vi "Read Next PNG Chunk.vi"(8 "error in (no error)":errorcluster, 11 "Byte Stream File in":refnum<file>) -> (0 "error out":errorcluster, 1 "data":u8[](array[numeric]), 2 "Type":string, 3 "Byte Stream File out":refnum<file>, 4 "CRC":u32, 5 "Length":u32)   [LabVIEW 2021, in "Files.lvlib"]
uses:
  Files.lvlib
  93311296-cc19-459f-8a29-a5908e25dff8.vi
  d1c91a06-6000-4e7e-a644-8d6add85a8ab.vi
  93311296-cc19-459f-8a29-a5908e25dff8.vi/539bd7ec-d9e8-460f-a56d-a449b4a86a5e.vi
  d1c91a06-6000-4e7e-a644-8d6add85a8ab.vi/539bd7ec-d9e8-460f-a56d-a449b4a86a5e.vi
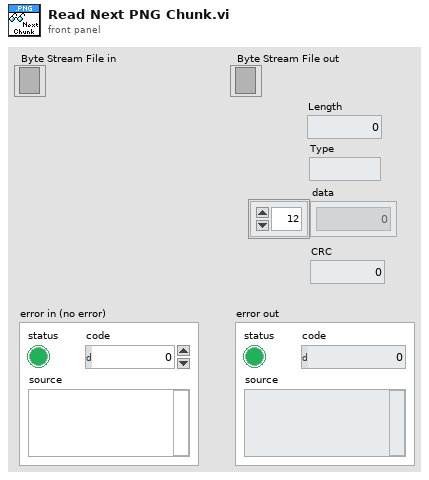
[diagram p1: front panel]
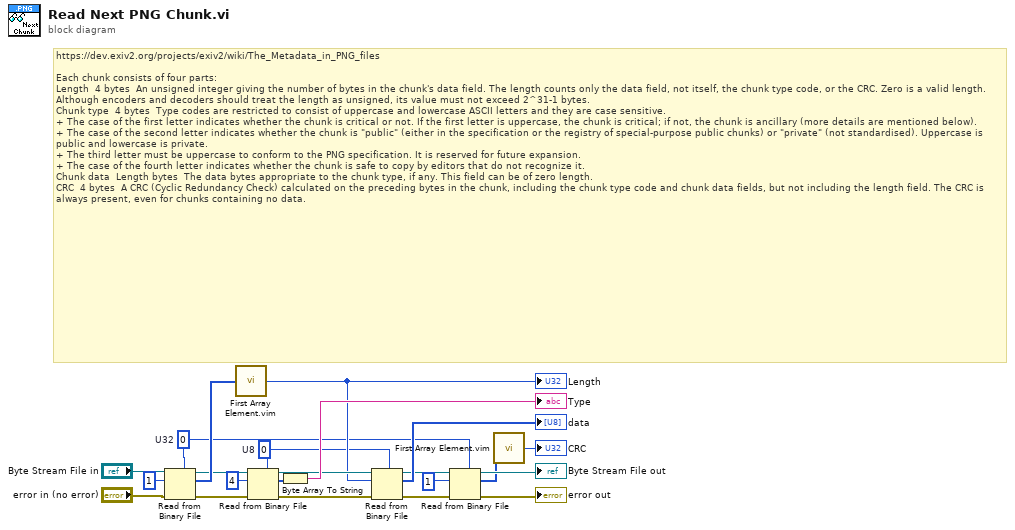
[diagram p0: block diagram]
diagram:
  w9 = u8 0  # U8
  w3 = u32 0  # U32
  # "https://dev.exiv2.org/projects/exiv2/wiki/The_Metadata_in_PNG_files\n\nEach chunk consists of four parts:\nLength \t4 bytes \tAn unsigned integer giving the number of bytes in the chunk's data field. The length counts only the data field, not itself, the chunk type code, or the CRC. Zero is a valid length. Although encoders and decoders should treat the length as unsigned, its value must not exceed 2^31-1 bytes.\nChunk type \t4 bytes \tType codes are restricted to consist of uppercase and lowercase ASCII letters and they are case sensitive.\n+ The case of the first letter indicates whether the chunk is critical or not. If the first letter is uppercase, the chunk is critical; if not, the chunk is ancillary (more details are mentioned below).\n+ The case of the second letter indicates whether the chunk is \"public\" (either in the specification or the registry of special-purpose public chunks) or \"private\" (not standardised). Uppercase is public and lowercase is private.\n+ The third letter must be uppercase to conform to the PNG specification. It is reserved for future expansion.\n+ The case of the fourth letter indicates whether the chunk is safe to copy by editors that do not recognize it.\nChunk data \tLength bytes \tThe data bytes appropriate to the chunk type, if any. This field can be of zero length.\nCRC \t4 bytes \tA CRC (Cyclic Redundancy Check) calculated on the preceding bytes in the chunk, including the chunk type code and chunk data fields, but not including the length field. The CRC is always present, even for chunks containing no data."
  n1 = Read from Binary File(5:w3, 8:"error in (no error)", 10:1 ("count (1)"), 11:"Byte Stream File in") -> (0:w19:errorcluster, 2:w18:u32[], 3:w16:refnum<file>)  [unwired: 2 in, 1 out]
  n2 = call "First Array Element.vim"("Array"=w18) -> ("First Element"=w10:u32)  [unwired: 8 in]
  "Length" <- w10
  n3 = Read from Binary File(5:w9, 8:w19, 10:4 ("count (1)"), 11:w16) -> (0:w17:errorcluster, 2:w14:u8[], 3:w11:refnum<file>)  [unwired: 2 in, 1 out]
  n4 = Byte Array To String(unsigned byte array=w14) -> (string=→"Type":string)
  n5 = Read from Binary File(5:w9, 8:w17, 10:w10, 11:w11) -> (0:w12:errorcluster, 2:→"data":u8[], 3:w6:refnum<file>)  [unwired: 2 in, 1 out]
  n6 = Read from Binary File(5:w3, 8:w12, 10:1 ("count (1)"), 11:w6) -> (0:→"error out":errorcluster, 2:w2:u32[], 3:→"Byte Stream File out":refnum<file>)  [unwired: 2 in, 1 out]
  n7 = call "First Array Element.vim"("Array"=w2) -> ("First Element"=→"CRC":u32)  [unwired: 8 in]
